vi "subFilterForRuleParsers.vi"(8 "error in (no error)":errorcluster, 9 "Addons":path[](array[path]), 11 "UIManager in":refnum<class "UIManager.lvclass">) -> (0 "error out":errorcluster, 3 "UIManager out":refnum<class "UIManager.lvclass">)   [LabVIEW 2020, in "UserInterface.lvlib" / "UIManager.lvclass"]
uses:
  UIManager.lvclass
  ExtensionInterfaces/IRuleFileParser/IRuleFileParser.lvclass
  8b2faf2b-35f3-477d-b08e-46dd3110fb1d.vi
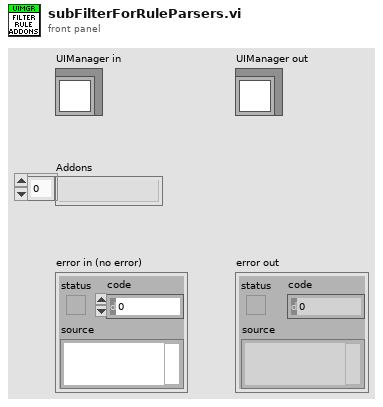
[diagram p1: front panel]
types:
  T1 = map{string, refnum<class "IRuleFileParser.lvclass">}
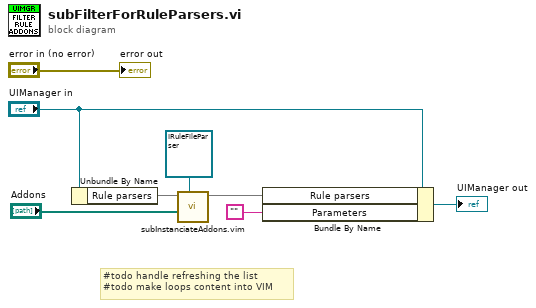
[diagram p0: block diagram]
diagram:
  # "#todo handle refreshing the list\n#todo make loops content into VIM"
  n1 = Unbundle By Name("UIManager in") -> ("Rule parsers"=w2:T1)
  n2 = call "subInstanciateAddons.vim"("Target object"=refnum<class "IRuleFileParser.lvclass"> refnum ("ExtensionInterfaces.lvlib:IRuleFileParser.lvclass"), "Addons"="Addons", "Addon map in"=w2) -> ("Addon map"=w4:T1)  [unwired: 8 in]
  n3 = Bundle By Name(cluster="UIManager in", "Rule parsers"=w4, "Parameters"="") -> (→"UIManager out":refnum<class "UIManager.lvclass">)
  "error out" <- "error in (no error)"
